vi "String to Double.vi"(8 "error in (no error)":errorcluster, 11 "String to Convert":string) -> (0 "error out":errorcluster, 3 "Double Value":dbl format="%#.6g")   [LabVIEW 2023, in "HAF.lvlib"]
doc: "Given a String representation of a Floating Point, returns it as a Double. If it can't be converted to a Double, an error is raised."
uses:
  HAF.lvlib
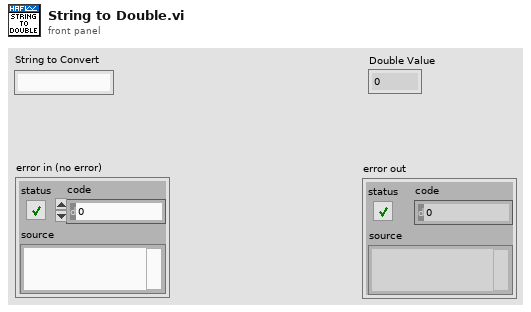
[diagram p1: front panel]
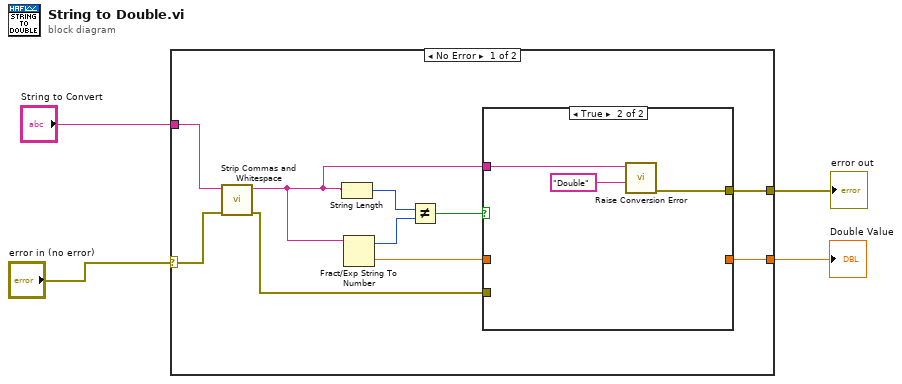
[diagram p0: block diagram]
diagram:
  n1 = case shown="No Error" "error in (no error)" {
    selector: "error in (no error)" -> [w13 w20]
    tunnel: "String to Convert" -> [w14 _]
    tunnel: [w7 w20] -> w2
    tunnel: [w6 _] -> w1
    frame No Error {
      n2 = call "Strip Commas and Whitespace.vi"("error in (no error)"=w13, "String to Strip"=w14) -> ("error out"=w5:errorcluster, "Clean String"=w9:string)  [unwired: 8 in]
      n3 = String Length(string=w9) -> (length=w12:i32)
      n4 = Fract/Exp String To Number(string=w9) -> (offset past number=w11:i32, number=w8:dbl)  [unwired: 3 in]
      n5 = Not Equal?(x=w12, y=w11) -> (x != y?=w10:bool)
      n6 = case shown="True" w10 {
        tunnel: w9 -> [_ w18]
        tunnel: w8 -> [w16 _]
        tunnel: [w15 w17] -> w7
        tunnel: [w16 _] -> w6
        tunnel: w5 -> [w15 _]
        frame False {
        }
        frame True {
          n7 = call "Raise Conversion Error.vi"("Data Type Attempted"="Double", "String in Error"=w18) -> ("error out"=w17:errorcluster)  [unwired: 9 in]
        }
      }
    }
    frame Error {
    }
  }
  "Double Value" <- w1
  "error out" <- w2
